vi "update_graphsSD.vi"(6 "wavelengths":dbl[](array[numeric]), 7 "timedelays":dbl[](array[numeric]), 8 "data":dbl[][](array[numeric]), 9 "IntensityGraph in":refnum<vi>) -> (0 "From wave":dbl, 1 "Kinetics":cluster{"timedelay":dbl[], dbl[]}[](array[cluster]), 2 "Spectrum":cluster{"Unités abscisse":dbl[], dbl[]}[](array[cluster]), 3 "To time":dbl, 4 "To wave":dbl, 5 "From  time":dbl)   [LabVIEW 2015]
types:
  T1 = cluster{"Max Y pixel":i32, "Min Y pixel":i32, "Max X pixel":i32, "Min X pixel":i32}
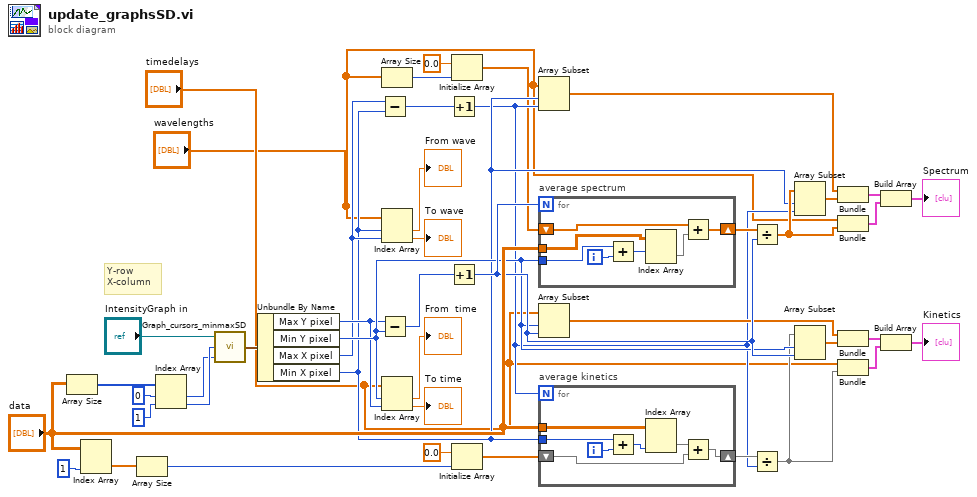
[diagram p0: block diagram]
diagram:
  # "Y-row\nX-column"
  n1 = Array Size(array="data") -> (size(s)=w17:i32[])
  n2 = Index Array(array="data", index (col)=1 ("disabled index (col)")) -> (element=w4:dbl[])  [unwired: 1 in]
  n3 = Array Size(array=w4) -> (size(s)=w6:i32)
  n4 = Index Array(array=w17, index #1=0 ("index"), index #2=1 ("index")) -> (element #1=w20:i32, element #2=w21:i32)
  n5 = call "Graph_cursors_minmaxSD.vi"("Max Y pixel"=w20, "Max X pixel"=w21, "GRAPH EXPERIMENTAL DATA"="IntensityGraph in") -> ("max/min XY pixels"=w22:T1)
  n6 = Unbundle By Name(w22) -> ("Max Y pixel"=w36:i32, "Min Y pixel"=w42:i32, "Max X pixel"=w34:i32, "Min X pixel"=w15:i32)
  n7 = Subtract(x=w34, y=w15) -> (x-y=w25:i32)
  n8 = Subtract(x=w36, y=w42) -> (x-y=w24:i32)
  n9 = Array Size(array="wavelengths") -> (size(s)=w7:i32)
  n10 = Index Array(array="wavelengths", index #1=w15, index #2=w34) -> (element #1=→"From wave":dbl, element #2=→"To wave":dbl)
  n11 = Index Array(array="timedelays", index #1=w42, index #2=w36) -> (element #1=→"From  time":dbl, element #2=→"To time":dbl)
  n12 = Increment(x=w25) -> (x+1=w14:i32)
  n13 = Increment(x=w24) -> (x+1=w43:i32)
  n14 = Initialize Array(0.0 ("element"), w7) -> (w9:dbl[])
  n15 = Initialize Array(0.0 ("element"), w6) -> (w3:dbl[])
  n16 = Array Subset(array="wavelengths", index=w15, length=w14) -> (w40:dbl[])
  n17 = for "average spectrum" {
    N: w43 -> [_]
    shift-right: [w51] -> w37
    shift-left: w9 -> [w48]
    tunnel: w42 -> [w49]
    tunnel: "data" -> [w47]
    i -> [w50]
    n18 = Add(x=w49, y=w50) -> (x+y=w46:i32)
    n19 = Index Array(array=w47, index (row)=w46) -> (element=w45:dbl[])  [unwired: 1 in]
    n20 = Add(x=w48, y=w45) -> (x+y=w51:dbl[])
  }
  n21 = Array Subset(array="timedelays", index=w42, length=w43) -> (w23:dbl[])
  n22 = for "average kinetics" {
    N: w14 -> [_]
    tunnel: "data" -> [w58]
    tunnel: w15 -> [w56]
    shift-right: [w52] -> w26
    shift-left: w3 -> [w53]
    i -> [w57]
    n23 = Add(x=w56, y=w57) -> (x+y=w55:i32)
    n24 = Index Array(array=w58, index (col)=w55) -> (element=w54:dbl[])  [unwired: 1 in]
    n25 = Add(x=w54, y=w53) -> (x+y=w52:dbl[])
  }
  n26 = Divide(x=w37, y=w43) -> (x/y=w39:dbl[])
  n27 = Divide(x=w26, y=w14) -> (x/y=w27:dbl[])
  n28 = Array Subset(array=w39, index=w15, length=w14) -> (w41:dbl[])
  n29 = Array Subset(array=w27, index=w42, length=w43) -> (w28:dbl[])
  n30 = Bundle(w40, w41) -> (w11:cluster{dbl[], dbl[]})  [unwired: 1 in]
  n31 = Bundle("wavelengths"="wavelengths", w39) -> (w10:cluster{"wavelengths":dbl[], dbl[]})  [unwired: 1 in]
  n32 = Bundle(w23, w28) -> (w12:cluster{dbl[], dbl[]})  [unwired: 1 in]
  n33 = Bundle("timedelays"="timedelays", w27) -> (w13:cluster{"timedelays":dbl[], dbl[]})  [unwired: 1 in]
  n34 = Build Array(w11, w10) -> (→"Spectrum":cluster{"wavelengths":dbl[], dbl[]}[])
  n35 = Build Array(w12, w13) -> (→"Kinetics":cluster{"timedelays":dbl[], dbl[]}[])
